vi "Write Depth Data.vi"(8 "error in (no error)":errorcluster, 10 "Depth Data":T1, 11 "Depth Data Message in":refnum<class "Depth Data Message.lvclass">) -> (0 "error out":errorcluster, 3 "Depth Data Message out":refnum<class "Depth Data Message.lvclass">)   [LabVIEW 2015, in "RDS Child Messages.lvlib" / "Depth Data Message.lvclass"]
uses:
  Depth Data Message.lvclass
  Depth Data.ctl
  Depth Data Message.lvclass/Depth Data Message.ctl
  RDS Child Messages.lvlib
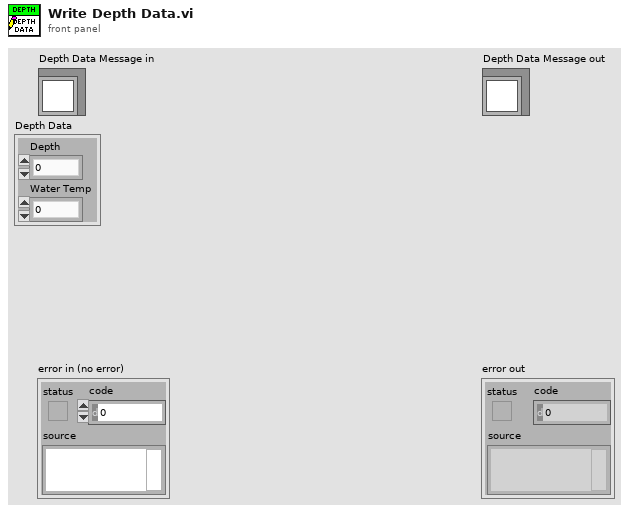
[diagram p1: front panel]
types:
  T1 = typedef "RDS Child Messages.lvlib/Depth Data.ctl" = cluster{"Depth":sgl, "Water Temp":i8}
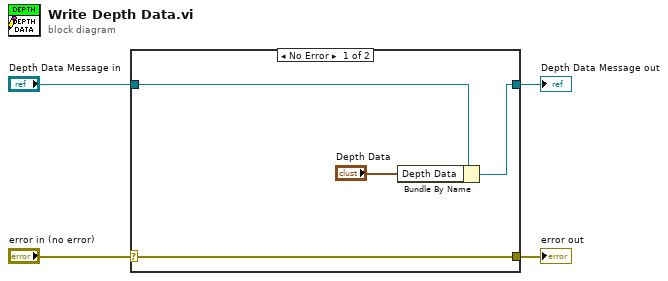
[diagram p0: block diagram]
diagram:
  n1 = case shown="No Error" "error in (no error)" {
    selector: "error in (no error)" -> [w8 w9]
    tunnel: [w8 w9] -> w3
    tunnel: [w6 w10] -> w1
    tunnel: "Depth Data Message in" -> [w7 w10]
    frame No Error {
      n2 = Bundle By Name(cluster=w7, "Depth Data"="Depth Data") -> (w6:refnum<class "Depth Data Message.lvclass">)
    }
    frame Error {
    }
  }
  "error out" <- w3
  "Depth Data Message out" <- w1
